vi "FEAT.vi"(8 "error in (no error)":errorcluster, 11 "FTP in":refnum<class "FTP.lvclass">) -> (0 "error out":errorcluster, 3 "FTP out":refnum<class "FTP.lvclass">)   [LabVIEW 2013, in "FTP.lvlib" / "FTP.lvclass"]
uses:
  FTP.lvclass
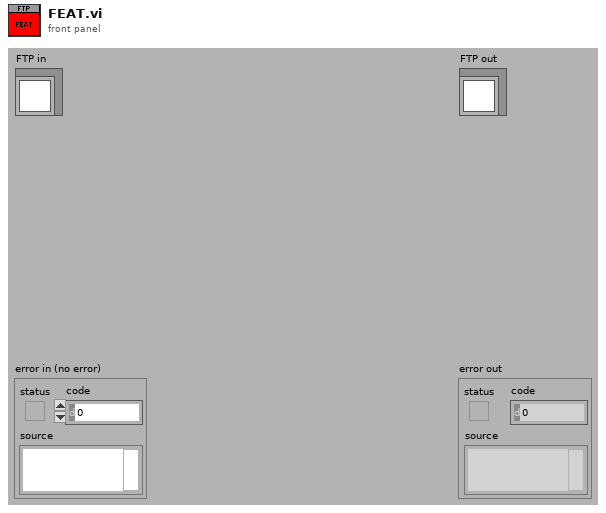
[diagram p1: front panel]
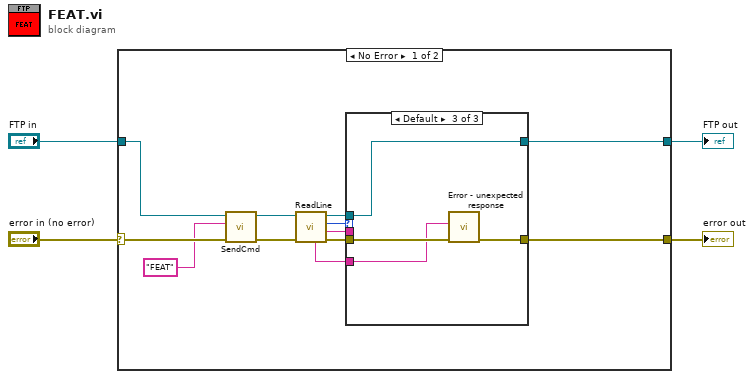
[diagram p0: block diagram]
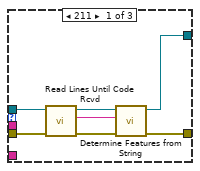
[diagram p2: hidden frame]
diagram:
  n1 = case shown="No Error" "error in (no error)" {
    selector: "error in (no error)" -> [w14 w31]
    tunnel: [w11 w31] -> w3
    tunnel: [w12 w30] -> w1
    tunnel: "FTP in" -> [w13 w30]
    frame No Error {
      n2 = call "SendCmd.vi"("error in (no error)"=w14, "cmd"="FEAT", "FTP in"=w13) -> ("error out"=w16:errorcluster, "FTP out"=w15:refnum<class "FTP.lvclass">)  [unwired: 7 in]
      n3 = call "ReadLine.vi"("error in (no error)"=w16, "FTP in"=w15) -> ("error out"=w7:errorcluster, "Line"=w6:string, "code"=w8:i32, "FTP out"=w9:refnum<class "FTP.lvclass">, "Full Line"=w5:string)  [unwired: 5 in]
      n4 = case shown="Default" w8 {
        tunnel: w9 -> [w22 w25 w29]
        tunnel: w7 -> [w23 w24 w28]
        tunnel: [w19 w24 w27] -> w11
        tunnel: [w18 w25 w29] -> w12
        tunnel: w6 -> [_ _ _]
        tunnel: w5 -> [_ _ w26]
        frame 211 {
          n5 = call "Read Lines Until Code Rcvd.vi"("error in (no error)"=w23, "FTP in"=w22) -> ("error out"=w21:errorcluster, "String"=w17:string, "FTP out"=w20:refnum<class "FTP.lvclass">)  [unwired: 7 in]
          n6 = call "Determine Features from String.vi"("error in (no error)"=w21, "Features"=w17, "FTP in"=w20) -> ("error out"=w19:errorcluster, "FTP out"=w18:refnum<class "FTP.lvclass">)  [unwired: 7 in]
        }
        frame 500 {
        }
        frame Default {
          n7 = call "Error - unexpected response.vi"("error in (no error)"=w28, "Full Response"=w26) -> ("error out"=w27:errorcluster)  [unwired: 9 in]
        }
      }
    }
    frame Error {
    }
  }
  "error out" <- w3
  "FTP out" <- w1
